vi "AB_Engine_Create_Preserve_Hierarchy_Destination.vi"(8 "error in (no error)":errorcluster, 9 "parentIndex in":i32, 10 "newPath":path, 11 "destinations in":refnum<class "AB_Destination.lvclass">[](array[class])) -> (0 "error out":errorcluster, 1 "destinationIndex out":i32, 3 "destination out":refnum<class "AB_Destination.lvclass">[](array[class]))   [LabVIEW 2020]
uses:
  <vilib>/AppBuilder/AB_Classes/Destination/AB_Destination.lvclass
  <vilib>/AppBuilder/AB_Classes/Destination/Dest_SubDirectory/AB_SubDirectory.ctl
  <vilib>/AppBuilder/AB_Classes/Destination/AB_Destination.ctl
  <vilib>/AppBuilder/AB_Classes/Destination/Dest_SubDirectory/AB_Dest_SubDir.lvclass
  e:/builds/penguin/labview/branches/2020/dev/dist/vi.lib/AppBuilder/AB_Classes/Destination/AB_Destination.lvclass
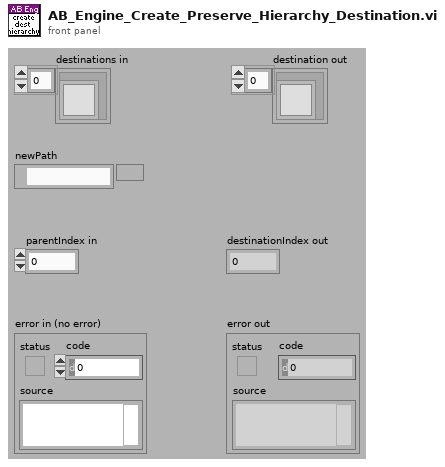
[diagram p1: front panel]
types:
  T1 = typedef "AB_SubDirectory.ctl" = cluster{"eng_parent":i32}
  T2 = typedef "AB_Destination.ctl" = cluster{"destName":string, "path":path, "libraryName":string, "preserveHierarchy":bool, "eng_inBuild":bool, "eng_libraryReference":refnum<vi>, "eng_restictAddToNewLibrary":bool}
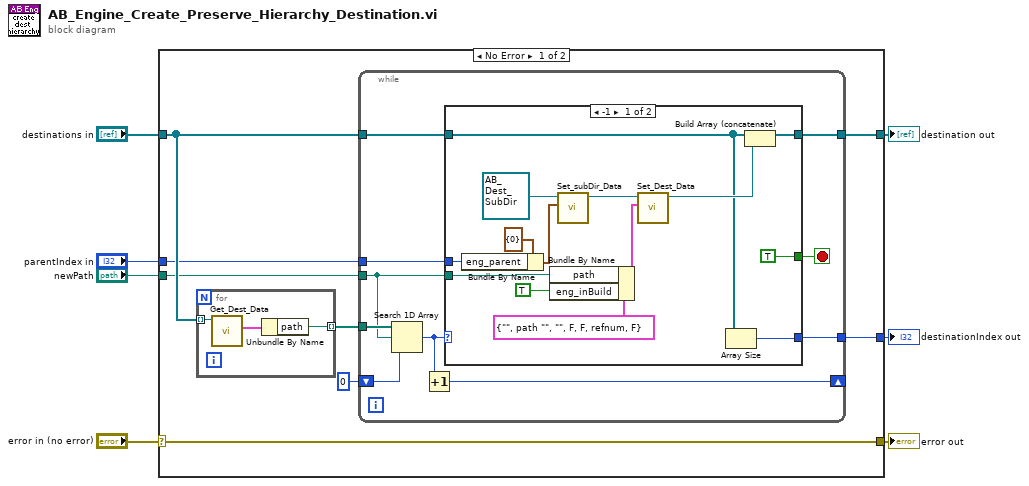
[diagram p0: block diagram]
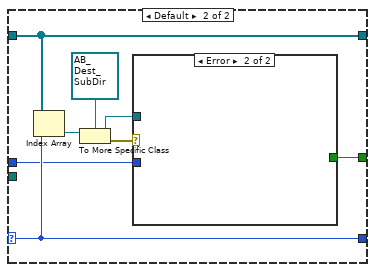
[diagram p2: hidden frame]
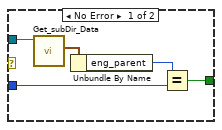
[diagram p3: hidden frame]
diagram:
  n1 = case shown="No Error" "error in (no error)" {
    selector: "error in (no error)" -> [w15 w57]
    tunnel: [w15 w57] -> w1
    tunnel: [w12 w56] -> w3
    tunnel: "destinations in" -> [w13 w56]
    tunnel: "newPath" -> [w11 _]
    tunnel: "parentIndex in" -> [w10 _]
    tunnel: [w9 _] -> w4
    frame No Error {
      n2 = for {
        tunnel: w13 -> [w54] mode=indexing
        tunnel: [w53] -> w14 mode=indexing
        n3 = call <vilib>:"Get_Dest_Data.vi"("Class in"=w54) -> ("destName"=w55:T2)  [unwired: 8 in, 2 out]
        n4 = Unbundle By Name(w55) -> ("path"=w53:path)
      }
      n5 = while {
        tunnel: w14 -> [w25]
        tunnel: w13 -> [w24]
        tunnel: [w23] -> w12
        tunnel: w11 -> [w22]
        tunnel: w10 -> [w21]
        tunnel: [w20] -> w9
        shift-right: [w17] -> _
        shift-left: 0 -> [w18]
        stop <- w16 stop-if-true
        n6 = Search 1D Array(1D array=w25, element=w22, start index (0)=w18) -> (index of element=w19:i32)
        n7 = Increment(x=w19) -> (x+1=w17:i32)
        n8 = case shown="-1" w19 {
          selector: w19 -> [_ w46]
          tunnel: [w34 w46] -> w20
          tunnel: w24 -> [w27 w47]
          tunnel: w22 -> [w36 _]
          tunnel: [w33 w47] -> w23
          tunnel: w21 -> [w29 w41]
          tunnel: [TRUE w40] -> w16
          frame -1 {
            n9 = Bundle By Name(cluster=T1 {"eng_parent"=0} ("data"), "eng_parent"=w29) -> (w28:T1)
            n10 = Bundle By Name(cluster=T2 {"destName"="", "path"=path "", "libraryName"="", "preserveHierarchy"=FALSE, "eng_inBuild"=FALSE, "eng_libraryReference"=refnum, "eng_restictAddToNewLibrary"=FALSE} ("destName"), "path"=w36, "eng_inBuild"=TRUE) -> (w39:T2)
            n11 = call <vilib>:"Set_subDir_Data.vi"("data"=w28, "AB_Dest_SubDir in"=refnum<class "AB_Dest_SubDir.lvclass"> refnum ("AB_Dest_SubDir.lvclass")) -> ("AB_Dest_SubDir out"=w31:refnum<class "AB_Dest_SubDir.lvclass">)  [unwired: 8 in, 1 out]
            n12 = call <vilib>:"Set_Dest_Data.vi"("destName"=w39, "Class in"=w31) -> ("Class out"=w38:refnum<class "AB_Dest_SubDir.lvclass">)  [unwired: 8 in, 1 out]
            n13 = Array Size(array=w27) -> (size(s)=w34:i32)
            n14 = Build Array (concatenate)(w27, w38) -> (w33:refnum<class "AB_Destination.lvclass">[])
          }
          frame Default {
            n15 = Index Array(array=w47, index=w46) -> (element=w45:refnum<class "AB_Destination.lvclass">)
            n16 = To More Specific Class(target class=refnum<class "AB_Dest_SubDir.lvclass"> refnum ("AB_Dest_SubDir.lvclass"), reference=w45) -> (specific class reference=w42:refnum<class "AB_Dest_SubDir.lvclass">, error out=w43:errorcluster)  [unwired: 1 in]
            n17 = case shown="Error" w43 {
              tunnel: w42 -> [w52 _]
              tunnel: w41 -> [w49 _]
              tunnel: [w48 _] -> w40
              frame No Error {
                n18 = call <vilib>:"Get_subDir_Data.vi"("AB_Dest_SubDir in"=w52) -> ("data"=w51:T1)  [unwired: 8 in, 2 out]
                n19 = Unbundle By Name(w51) -> ("eng_parent"=w50:i32)
                n20 = Equal?(x=w50, y=w49) -> (x = y?=w48:bool)
              }
              frame Error {
              }
            }
          }
        }
      }
    }
    frame Error {
    }
  }
  "error out" <- w1
  "destinationIndex out" <- w4
  "destination out" <- w3
